vi "CRYDrop Data in Diff Graph.vi"(10 "pGraph VI In":refnum<vi>, 11 "Graph Type":string) -> ()   [LabVIEW 2013]
uses:
  CRYData View Global.vi
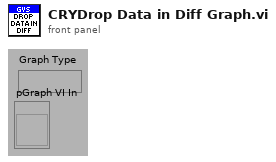
[diagram p1: front panel]
types:
  T1 = typedef "CRYDrag Graph.ctl" = cluster{"GraphType":string, "GraphData":variant}
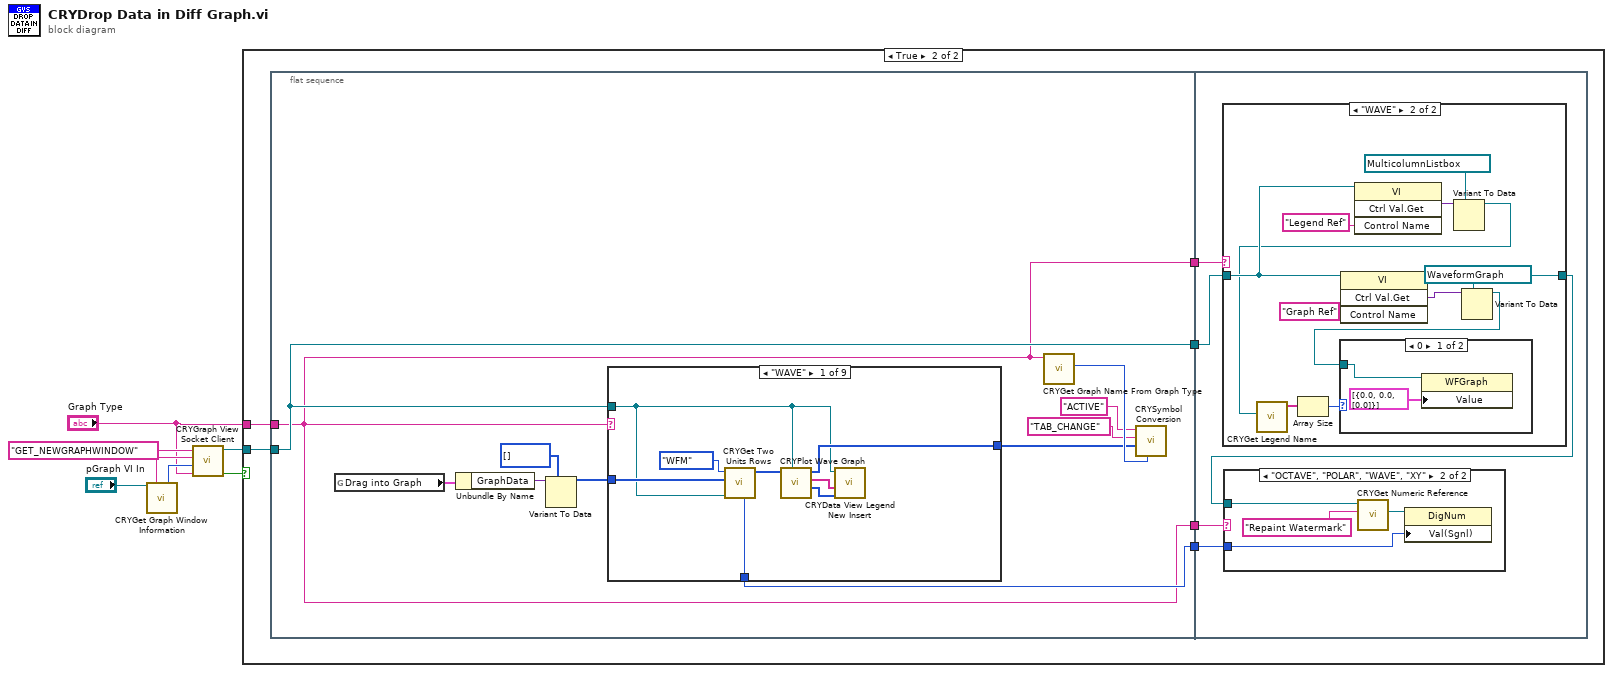
[diagram p0: block diagram]
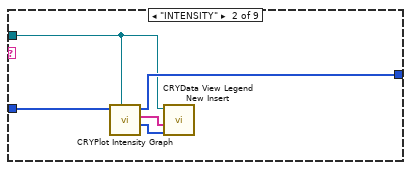
[diagram p3: hidden frame]
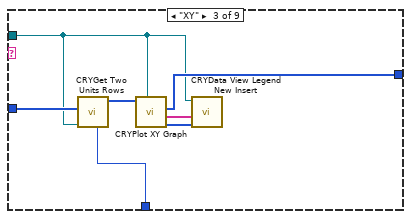
[diagram p4: hidden frame]
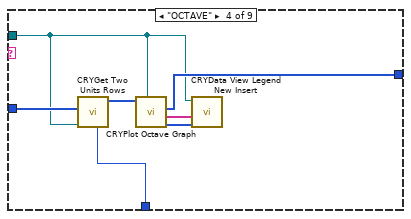
[diagram p5: hidden frame]
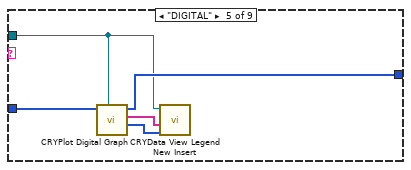
[diagram p6: hidden frame]
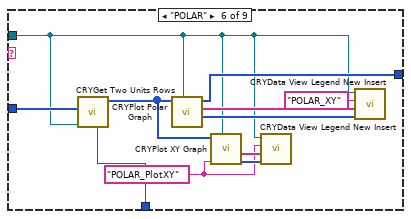
[diagram p7: hidden frame]
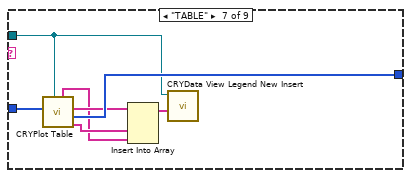
[diagram p8: hidden frame]
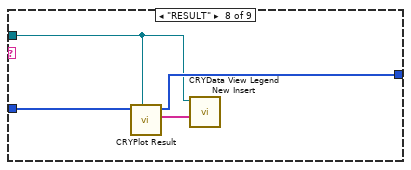
[diagram p9: hidden frame]
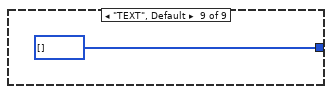
[diagram p10: hidden frame]
diagram:
  n1 = call "CRYGet Graph Window Information.vi"("pGraph VI In"="pGraph VI In") -> ("Queue Name Out"=w6:string, "Graph Number Out"=w5:i32)  [unwired: 4 in, 9 out]
  n2 = call "CRYGraph View Socket Client.vi"("sOption"="Graph Type", "nData"=w5, "sData"=w6, "sAction"="GET_NEWGRAPHWINDOW") -> ("bResult Out"=w2:bool, "pVI Out"=w3:refnum<vi>)  [unwired: 4 in, 2 out]
  n3 = case shown="True" w2 {
    tunnel: w3 -> [_ w9]
    tunnel: "Graph Type" -> [_ w13]
    frame False {
    }
    frame True {
      n4 = flat-sequence {
        tunnel: [w20] -> w12
        tunnel: [w18] -> w11
        tunnel: [w19] -> w10
        tunnel: w13 -> [w18]
        tunnel: w9 -> [w19]
        tunnel: [w18] -> w8
        tunnel: w12 -> [w84]
        tunnel: w11 -> [w83]
        tunnel: w10 -> [w82]
        tunnel: w8 -> [w80]
        frame #0 {
          n5 = global read "CRYData View Global.vi" "Drag into Graph"() -> (w17:T1)
          n6 = Unbundle By Name(w17) -> ("GraphData"=w16:variant)
          n7 = Variant To Data(type=i32[] [] ("Drag Rows"), Variant=w16) -> (data=w14:i32[])  [unwired: 1 in, 1 out]
          n8 = case shown="\"WAVE\"" w18 {
            tunnel: [w30 w35 w40 w47 w54 w67 w73 w78 i32[] [] ("Selected Rows Out")] -> w22
            tunnel: w14 -> [w28 w34 w44 w51 w53 w60 w74 w77 _]
            tunnel: [w26 _ w39 w46 _ w59 _ _ _] -> w20
            tunnel: w19 -> [w25 w33 w38 w45 w52 w57 w68 w75 _]
            frame "WAVE" {
              n9 = call "CRYGet Two Units Rows.vi"("pGraph VI In"=w25, "Old Rows In"=w28, "Type"=enum16{"Curves", "Values", "Results", "WFM"}."WFM") -> ("All Rows Out"=w27:i32[], "Two Units"=w26:i32)  [unwired: 2 in, 5 out]
              n10 = call "CRYPlot Wave Graph.vi"("pGraph VI In"=w25, "Selected Rows In"=w27) -> ("Color Info"=w31:u32[], "Curve Name"=w32:string[], "Selected Rows Out"=w30:i32[])  [unwired: 4 in, 3 out]
              n11 = call "CRYData View Legend New Insert.vi"("Color Array"=w31, "ItemName Array"=w32, "pGraph VI In"=w25) -> ()  [unwired: 2 in, 7 out]
            }
            frame "INTENSITY" {
              n12 = call "CRYPlot Intensity Graph.vi"("pGraph VI In"=w33, "Selected Rows In"=w34) -> ("Color Info"=w36:u32[], "Wave Names"=w37:string[], "All Rows Out"=w35:i32[])  [unwired: 6 in, 1 out]
              n13 = call "CRYData View Legend New Insert.vi"("Color Array"=w36, "ItemName Array"=w37, "pGraph VI In"=w33) -> ()  [unwired: 2 in, 7 out]
            }
            frame "XY" {
              n14 = call "CRYGet Two Units Rows.vi"("pGraph VI In"=w38, "Old Rows In"=w44) -> ("All Rows Out"=w43:i32[], "Two Units"=w39:i32)  [unwired: 3 in, 5 out]
              n15 = call "CRYPlot XY Graph.vi"("pGraph VI In"=w38, "Selected Rows In"=w43) -> ("Color Info"=w41:u32[], "Curve Name"=w42:string[], "All Rows Out"=w40:i32[])  [unwired: 4 in, 3 out]
              n16 = call "CRYData View Legend New Insert.vi"("Color Array"=w41, "ItemName Array"=w42, "pGraph VI In"=w38) -> ()  [unwired: 2 in, 7 out]
            }
            frame "OCTAVE" {
              n17 = call "CRYGet Two Units Rows.vi"("pGraph VI In"=w45, "Old Rows In"=w51) -> ("All Rows Out"=w50:i32[], "Two Units"=w46:i32)  [unwired: 3 in, 5 out]
              n18 = call "CRYPlot Octave Graph.vi"("pGraph VI In"=w45, "Selected Rows In"=w50) -> ("Color Info"=w48:u32[], "Curve Name"=w49:string[], "All Rows Out"=w47:i32[])  [unwired: 6 in, 1 out]
              n19 = call "CRYData View Legend New Insert.vi"("Color Array"=w48, "ItemName Array"=w49, "pGraph VI In"=w45) -> ()  [unwired: 2 in, 7 out]
            }
            frame "DIGITAL" {
              n20 = call "CRYPlot Digital Graph.vi"("pGraph VI In"=w52, "Selected Row In"=w53) -> ("Color Info"=w56:u32[], "Curve Name"=w55:string[], "Selected Row Out"=w54:i32[])  [unwired: 2 in, 5 out]
              n21 = call "CRYData View Legend New Insert.vi"("Color Array"=w56, "ItemName Array"=w55, "pGraph VI In"=w52) -> ()  [unwired: 2 in, 7 out]
            }
            frame "POLAR" {
              w58 = "POLAR_PlotXY" ("sOption")
              n22 = call "CRYGet Two Units Rows.vi"("pGraph VI In"=w57, "Old Rows In"=w60) -> ("All Rows Out"=w61:i32[], "Two Units"=w59:i32)  [unwired: 3 in, 5 out]
              n23 = call "CRYPlot Polar Graph.vi"("pGraph VI In"=w57, "Selected Rows In"=w61) -> ("Freq Color"=w65:u32[], "Freq Name"=w66:string[], "Selected Row Out"=w67:i32[])  [unwired: 4 in, 3 out]
              n24 = call "CRYPlot XY Graph.vi"("pGraph VI In"=w57, "sType"=w58, "Selected Rows In"=w61) -> ("Color Info"=w63:u32[], "Curve Name"=w64:string[])  [unwired: 5 in, 2 out]
              n25 = call "CRYData View Legend New Insert.vi"("Color Array"=w63, "ItemName Array"=w64, "sOption"=w58, "pGraph VI In"=w57) -> ()  [unwired: 1 in, 7 out]
              n26 = call "CRYData View Legend New Insert.vi"("Color Array"=w65, "ItemName Array"=w66, "sOption"="POLAR_XY", "pGraph VI In"=w57) -> ()  [unwired: 1 in, 7 out]
            }
            frame "TABLE" {
              n27 = call "CRYPlot Table.vi"("pGraph VI In"=w68, "Value Rows In"=w74) -> ("Value Name"=w70:string[], "Value Rows Out"=w73:i32[], "Curve Name"=w71:string[], "Result Name"=w69:string[])  [unwired: 4 in, 2 out]
              n28 = Insert Into Array(array=w71, new element #1=w70, new element #2=w69) -> (w72:string[])  [unwired: 1 in]
              n29 = call "CRYData View Legend New Insert.vi"("ItemName Array"=w72, "pGraph VI In"=w68) -> ()  [unwired: 3 in, 7 out]
            }
            frame "RESULT" {
              n30 = call "CRYPlot Result.vi"("pGraph VI In"=w75, "Old Rows In"=w77) -> ("Curve Name"=w76:string[], "Selected Rows Out"=w78:i32[])  [unwired: 4 in, 4 out]
              n31 = call "CRYData View Legend New Insert.vi"("ItemName Array"=w76, "pGraph VI In"=w75) -> ()  [unwired: 3 in, 7 out]
            }
            frame "TEXT", Default {
            }
          }
          n32 = call "CRYGet Graph Name From Graph Type.vi"("Graph Type"=w18) -> ("Type"=w24:enum16{"Curves", "Values", "Results", "WFM"})  [unwired: 9 in, 1 out]
          n33 = call "CRYSymbol Conversion.vi"("CurLib Tab Type"=w24, "nDatas"=w22, "sData"="TAB_CHANGE" ("sActin"), "sActin"="ACTIVE") -> ()  [unwired: 8 in]
        }
        frame #1 {
          n34 = case shown="\"WAVE\"" w80 {
            tunnel: w82 -> [w85 w88]
            tunnel: [w85 w91] -> w81
            frame "False", Default {
            }
            frame "WAVE" {
              n35 = invoke class="VI" method="Ctrl Val.Get"(reference=w88, "Control Name"="Graph Ref") -> (reference out=w91:refnum<vi>, "Get Control Value Variant"=w93:variant)  [unwired: 2 in, 2 out]
              n36 = invoke class="VI" method="Ctrl Val.Get"(reference=w88, "Control Name"="Legend Ref") -> ("Get Control Value Variant"=w89:variant)  [unwired: 2 in, 3 out]
              n37 = Variant To Data(type=refnum<vi> refnum ("GMListbox"), Variant=w89) -> (data=w86:refnum<vi>)  [unwired: 1 in, 1 out]
              n38 = call "CRYGet Legend Name.vi"("MCListbox Refnum"=w86) -> ("Names Out"=w96:string[])  [unwired: 2 in, 8 out]
              n39 = Array Size(array=w96) -> (size(s)=w97:i32)
              n40 = Variant To Data(type=refnum<vi> refnum ("WaveGraph Ref"), Variant=w93) -> (data=w92:refnum<vi>)  [unwired: 1 in, 1 out]
              n41 = case shown="0" w97 {
                tunnel: w92 -> [w99 _]
                frame 0 {
                  n42 = property class="WFGraph"(reference=w99, "Value"=cluster{"xo":dbl, "dx":dbl, dbl[]}[] [{"xo"=0.0, "dx"=0.0, [0.0]}] ("appended array")) -> ()  [unwired: 1 in, 2 out]
                }
                frame 1, Default {
                }
              }
            }
          }
          n43 = case shown="\"OCTAVE\", \"POLAR\", \"WAVE\", \"XY\"" w83 {
            tunnel: w81 -> [_ w101]
            tunnel: w84 -> [_ w100]
            frame Default {
            }
            frame "OCTAVE", "POLAR", "WAVE", "XY" {
              n44 = call "CRYGet Numeric Reference.vi"("Label Name"="Repaint Watermark" ("Control Name"), "VI Refnum"=w101) -> ("Numeric Ref Out"=w103:refnum<vi>)  [unwired: 9 out]
              n45 = property class="DigNum"(reference=w103, "Val(Sgnl)"=w100) -> ()  [unwired: 1 in, 2 out]
            }
          }
        }
      }
    }
  }
